vi "test_section_daqmx_task.vi"(8 "error in":errorcluster, 9 "Test Section Physical Channels":T1={"Vapor Mass Flow Current"="cDAQ1Mod1/ai10", "Vapor Line Density Current"="cDAQ1Mod1/ai11", "Liquid Mass Flow Current"="cDAQ1Mod1/ai8", "Liquid Line Density Current"="cDAQ1Mod1/ai9", "Vapor Tank Pressure"="cDAQ1Mod1/ai3", "Liquid Tank Pressure"="cDAQ1Mod1/ai6", "Separator Pressure"="cDAQ1Mod1/ai2", "Liquid Inlet Pressure"="cDAQ1Mod1/ai4", "Vapor Inlet Pressure"="cDAQ1Mod1/ai0", "Vapor Tank Temperature"="cDAQ1Mod1/ai1", "Vapor Inlet Temperature"="cDAQ1Mod6/ai2", "Liquid Tank Temperature"="cDAQ1Mod6/ai0", "Liquid Inlet Temperature"="cDAQ1Mod6/ai3", "Separator Temperature"="cDAQ1Mod6/ai4", "Lower Dev Section Pressure"="cDAQ1Mod6/ai1", "Test Section Temperature"="cDAQ1Mod1/ai5", "Upper Dev Section Temperature"="cDAQ1Mod1/ai12", "Upper Dev Section Pressure"="cDAQ1Mod6/ai9", "Atmospheric Pressure"="cDAQ1Mod5/ai7", "Mixing Tee dP"="cDAQ1Mod6/ai5", "PG inlet-Mixing Tee Pressure"="cDAQ1Mod6/ai5", "Test Section Pressure"="cDAQ1Mod5/ai7", "PG inlet-Mixing Tee Temperature"="cDAQ1Mod6/ai5"}) -> (0 "error out":errorcluster, 3 "task out":refnum<k21>)   [LabVIEW 2017]
uses:
  Input Channel Lists/test_section_physical_channels.ctl
  <vilib>/DAQmx/create/channels.llb/DAQmx Create Channel (AI-Current-Basic).vi
  <vilib>/DAQmx/create/channels.llb/DAQmx Create Channel (AI-Voltage-Basic).vi
  <vilib>/DAQmx/create/channels.llb/DAQmx Create Channel (AI-Temperature-Thermocouple).vi
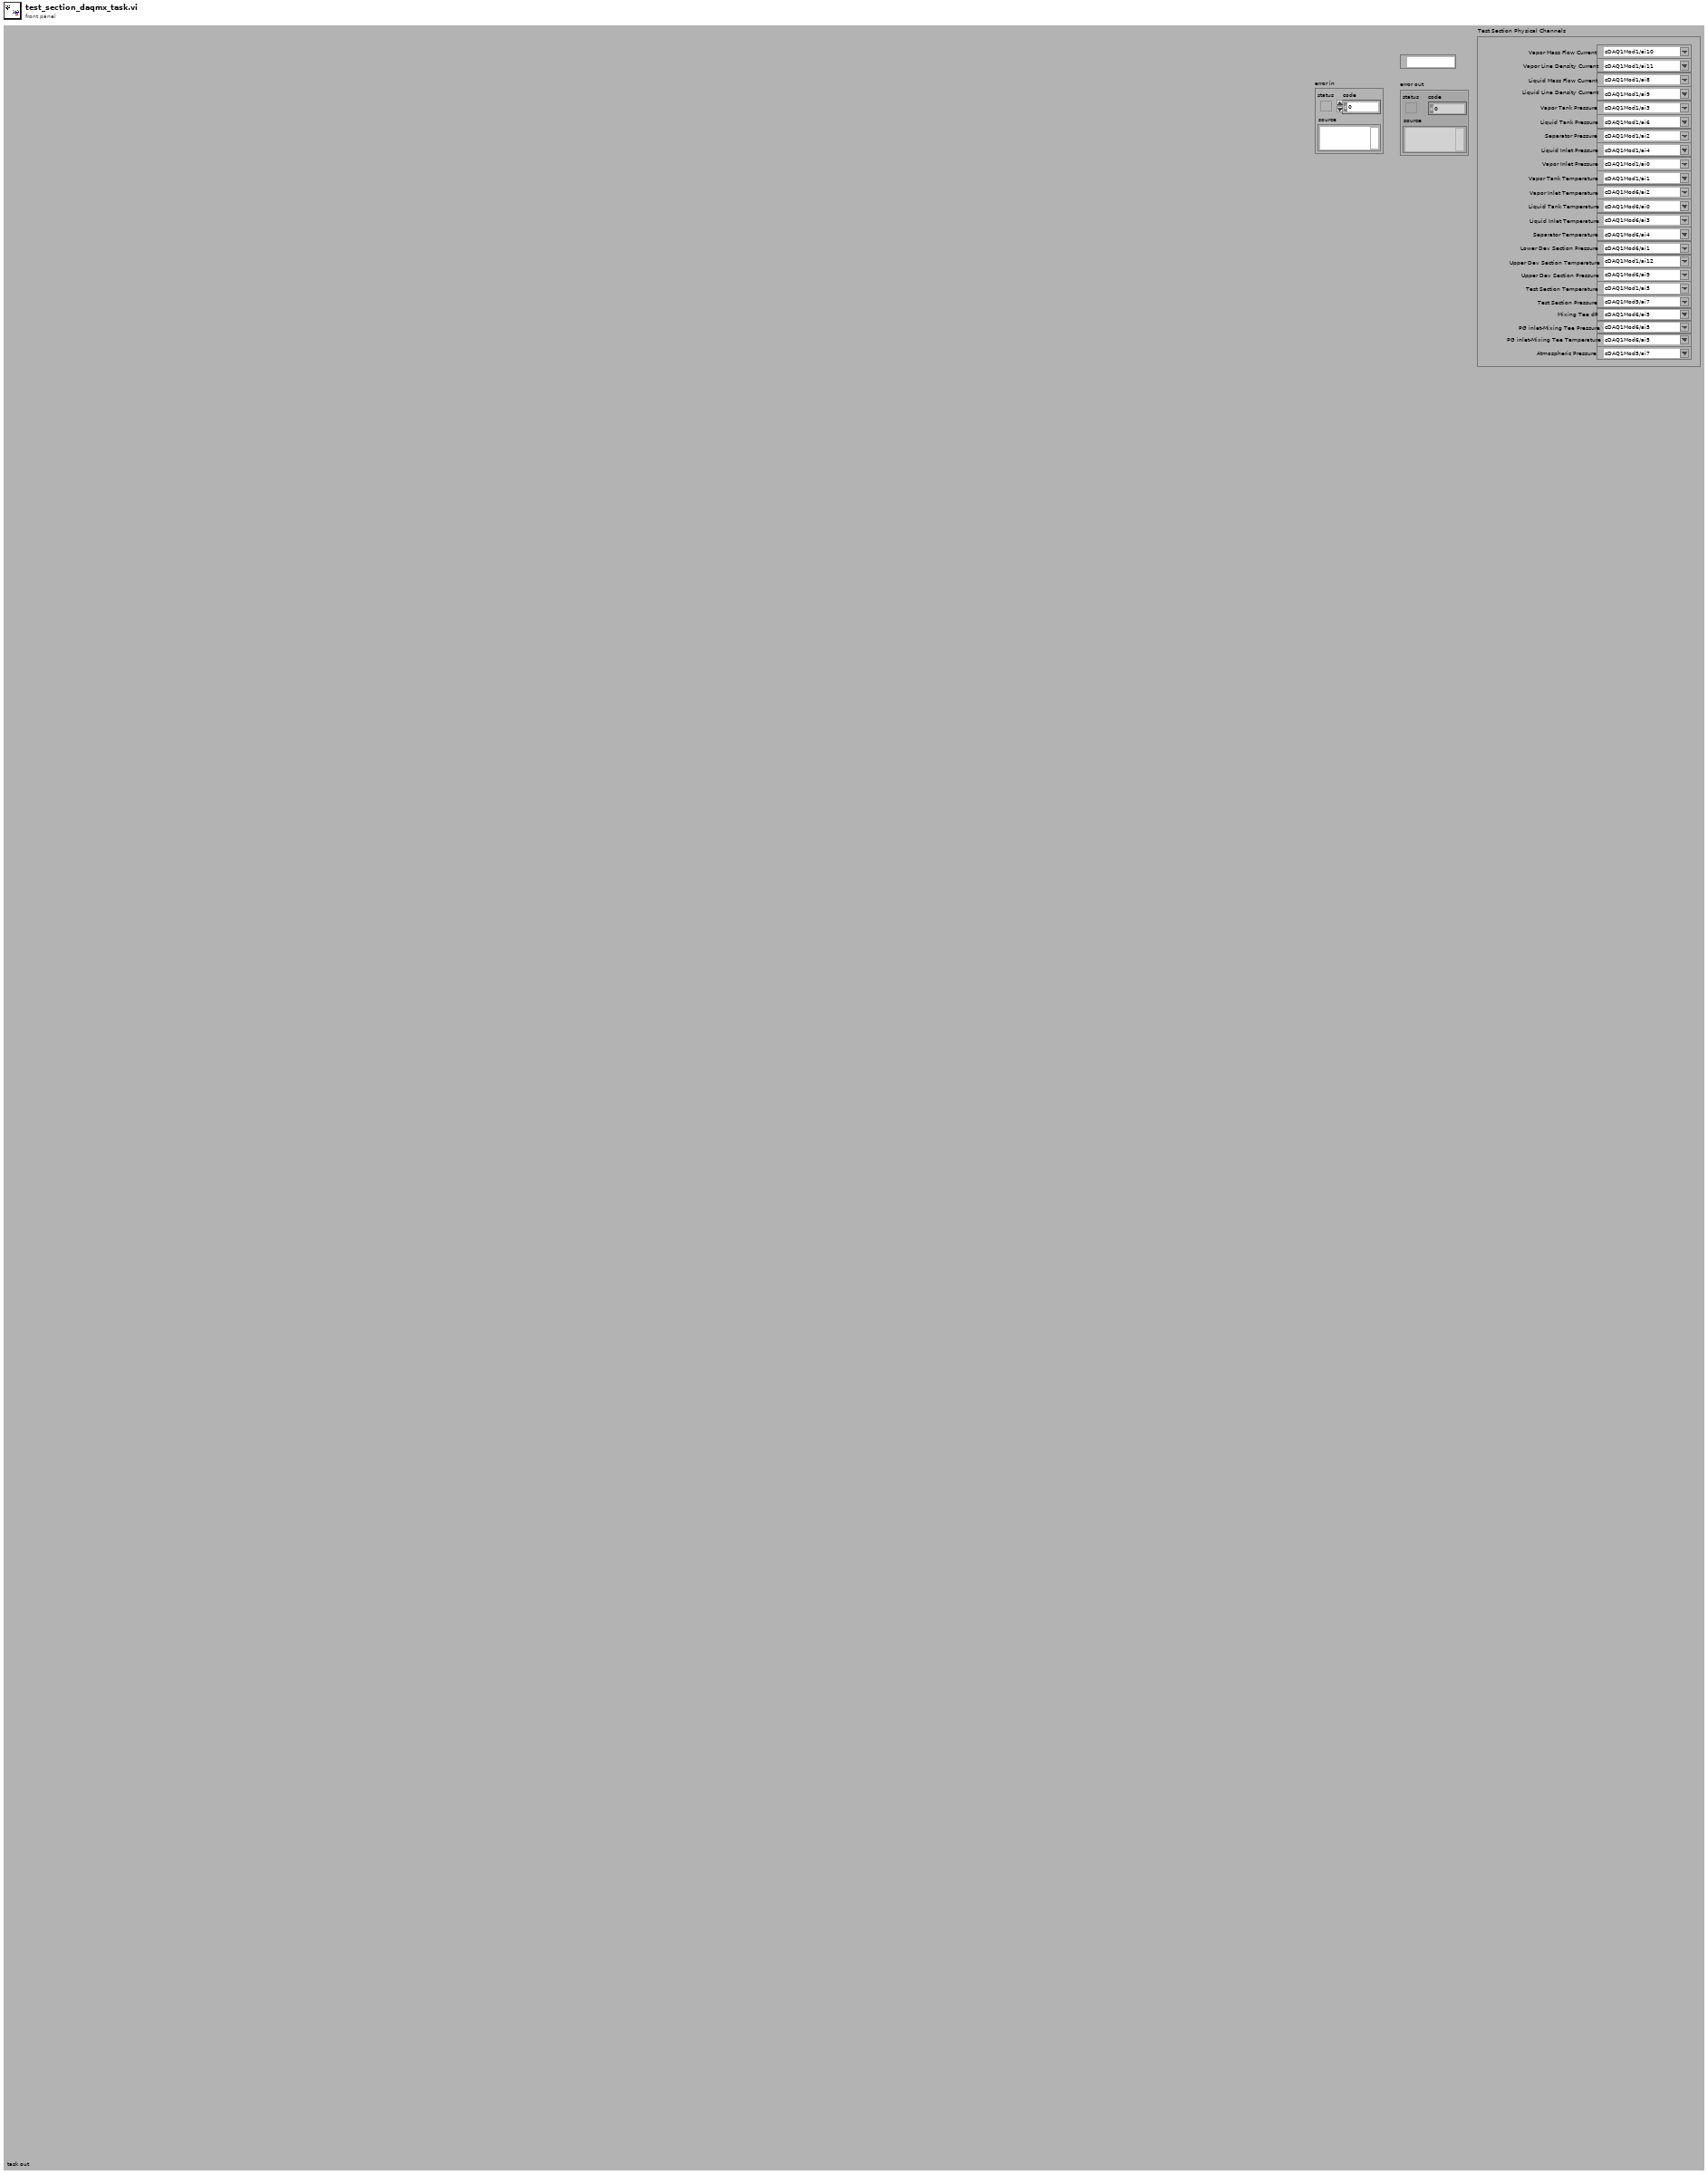
[diagram p1: front panel]
types:
  T1 = typedef "test_section_physical_channels.ctl" = cluster{"Vapor Mass Flow Current":tag, "Vapor Line Density Current":tag, "Liquid Mass Flow Current":tag, "Liquid Line Density Current":tag, "Vapor Tank Pressure":tag, "Liquid Tank Pressure":tag, "Separator Pressure":tag, "Liquid Inlet Pressure":tag, "Vapor Inlet Pressure":tag, "Vapor Tank Temperature":tag, "Vapor Inlet Temperature":tag, "Liquid Tank Temperature":tag, "Liquid Inlet Temperature":tag, "Separator Temperature":tag, "Lower Dev Section Pressure":tag, "Test Section Temperature":tag, "Upper Dev Section Temperature":tag, "Upper Dev Section Pressure":tag, "Atmospheric Pressure":tag, "Mixing Tee dP":tag, "PG inlet-Mixing Tee Pressure":tag, "Test Section Pressure":tag, "PG inlet-Mixing Tee Temperature":tag}
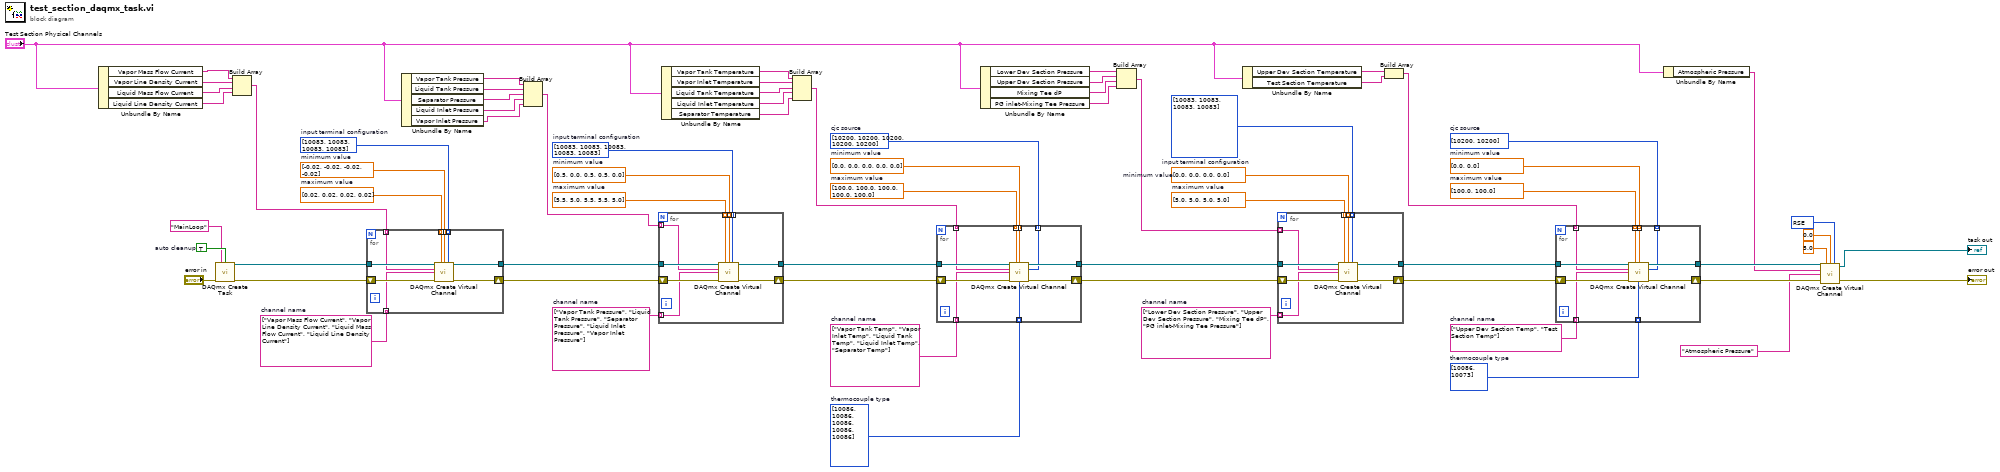
[diagram p0: block diagram]
diagram:
  w4 = 10083 items=["Default"=-1, "RSE"=10083, "NRSE"=10078, "Differential"=10106, "Pseudodifferential"=12529] ("input terminal configuration")
  w39 = i32[] [10086, 10073] items=["J"=10072, "K"=10073, "N"=10077, "R"=10082, "S"=10085, "T"=10086, "B"=10047, "E"=10055]  # thermocouple type
  w38 = string[] ["Upper Dev Section Temp", "Test Section Temp"]  # channel name
  w40 = dbl[] [100.0, 100.0]  # maximum value
  w41 = dbl[] [0.0, 0.0]  # minimum value
  w37 = u32[] [10200, 10200] items=["Internal"=10200, "Constant Value"=10116, "Channel"=10113]  # cjc source
  w44 = string[] ["Lower Dev Section Pressure", "Upper Dev Section Pressure", "Mixing Tee dP", "PG inlet-Mixing Tee Pressure"]  # channel name
  w45 = dbl[] [5.0, 5.0, 5.0, 5.0]  # maximum value
  w46 = dbl[] [0.0, 0.0, 0.0, 0.0]  # minimum value
  w47 = i32[] [10083, 10083, 10083, 10083] items=["default"=-1, "RSE"=10083, "NRSE"=10078, "Differential"=10106, "Pseudodifferential"=12529]  # input terminal configuration
  w52 = i32[] [10086, 10086, 10086, 10086, 10086] items=["J"=10072, "K"=10073, "N"=10077, "R"=10082, "S"=10085, "T"=10086, "B"=10047, "E"=10055]  # thermocouple type
  w51 = string[] ["Vapor Tank Temp", "Vapor Inlet Temp", "Liquid Tank Temp", "Liquid Inlet Temp", "Separator Temp"]  # channel name
  w53 = dbl[] [100.0, 100.0, 100.0, 100.0, 100.0]  # maximum value
  w54 = dbl[] [0.0, 0.0, 0.0, 0.0, 0.0]  # minimum value
  w49 = u32[] [10200, 10200, 10200, 10200, 10200] items=["Internal"=10200, "Constant Value"=10116, "Channel"=10113]  # cjc source
  w57 = string[] ["Vapor Tank Pressure", "Liquid Tank Pressure", "Separator Pressure", "Liquid Inlet Pressure", "Vapor Inlet Pressure"]  # channel name
  w58 = dbl[] [5.5, 5.0, 5.5, 5.5, 5.0]  # maximum value
  w59 = dbl[] [0.5, 0.0, 0.5, 0.5, 0.0]  # minimum value
  w60 = i32[] [10083, 10083, 10083, 10083, 10083] items=["default"=-1, "RSE"=10083, "NRSE"=10078, "Differential"=10106, "Pseudodifferential"=12529]  # input terminal configuration
  w63 = string[] ["Vapor Mass Flow Current", "Vapor Line Density Current", "Liquid Mass Flow Current", "Liquid Line Density Current"]  # channel name
  w64 = dbl[] [0.02, 0.02, 0.02, 0.02]  # maximum value
  w65 = dbl[] [-0.02, -0.02, -0.02, -0.02]  # minimum value
  w66 = i32[] [10083, 10083, 10083, 10083] items=["default"=-1, "RSE"=10083, "NRSE"=10078, "Differential"=10106, "Pseudodifferential"=12529]  # input terminal configuration
  w68 = TRUE  # auto cleanup
  n1 = Unbundle By Name("Test Section Physical Channels") -> ("Vapor Mass Flow Current"=w35:tag, "Vapor Line Density Current"=w34:tag, "Liquid Mass Flow Current"=w33:tag, "Liquid Line Density Current"=w32:tag)
  n2 = call <vilib>:"DAQmx Create Task.vi"("new task name"="MainLoop", "auto cleanup"=w68, "error in"="error in") -> ("task out"=w67:refnum<k21>, "error out"=w69:errorcluster)  [unwired: 11 in]
  n3 = Build Array(w35, w34, w33, w32) -> (w31:tag[])
  n4 = for {
    tunnel: w67 -> [w76]
    tunnel: w66 -> [w79] mode=indexing
    tunnel: w65 -> [w78] mode=indexing
    tunnel: w64 -> [w77] mode=indexing
    tunnel: w63 -> [w72] mode=indexing
    tunnel: w31 -> [w71] mode=indexing
    tunnel: [w74] -> w61
    shift-right: [w73] -> w62
    shift-left: w69 -> [w75]
    n5 = call-poly <vilib>:"DAQmx Create Virtual Channel.vi"("task in"=w76, "maximum value"=w77, "minimum value"=w78, "input terminal configuration"=w79, "physical channels"=w71, "name to assign"=w72, "error in"=w75) -> ("task out"=w74:refnum<k21>, "error out"=w73:errorcluster)  [unwired: 7 in]
  }
  n6 = Unbundle By Name("Test Section Physical Channels") -> ("Vapor Tank Pressure"=w27:tag, "Liquid Tank Pressure"=w28:tag, "Separator Pressure"=w29:tag, "Liquid Inlet Pressure"=w30:tag, "Vapor Inlet Pressure"=w21:tag)
  n7 = Build Array(w27, w28, w29, w30, w21) -> (w20:tag[])
  n8 = for {
    tunnel: w61 -> [w85]
    tunnel: w60 -> [w86] mode=indexing
    tunnel: w59 -> [w87] mode=indexing
    tunnel: w58 -> [w88] mode=indexing
    tunnel: w57 -> [w81] mode=indexing
    tunnel: w20 -> [w80] mode=indexing
    tunnel: [w83] -> w55
    shift-right: [w82] -> w56
    shift-left: w62 -> [w84]
    n9 = call-poly <vilib>:"DAQmx Create Virtual Channel.vi"("task in"=w85, "maximum value"=w88, "minimum value"=w87, "input terminal configuration"=w86, "physical channels"=w80, "name to assign"=w81, "error in"=w84) -> ("task out"=w83:refnum<k21>, "error out"=w82:errorcluster)  [unwired: 7 in]
  }
  n10 = Unbundle By Name("Test Section Physical Channels") -> ("Vapor Tank Temperature"=w26:tag, "Vapor Inlet Temperature"=w25:tag, "Liquid Tank Temperature"=w24:tag, "Liquid Inlet Temperature"=w23:tag, "Separator Temperature"=w19:tag)
  n11 = Build Array(w26, w25, w24, w23, w19) -> (w18:tag[])
  n12 = for {
    tunnel: w55 -> [w96]
    tunnel: w54 -> [w97] mode=indexing
    tunnel: w53 -> [w98] mode=indexing
    tunnel: w52 -> [w89] mode=indexing
    tunnel: w51 -> [w92] mode=indexing
    tunnel: w18 -> [w91] mode=indexing
    tunnel: [w94] -> w48
    tunnel: w49 -> [w90] mode=indexing
    shift-right: [w93] -> w50
    shift-left: w56 -> [w95]
    n13 = call-poly <vilib>:"DAQmx Create Virtual Channel.vi"("task in"=w96, "maximum value"=w98, "minimum value"=w97, "physical channels"=w91, "cjc source"=w90, "name to assign"=w92, "error in"=w95, "thermocouple type"=w89) -> ("task out"=w94:refnum<k21>, "error out"=w93:errorcluster)  [unwired: 6 in]
  }
  n14 = Unbundle By Name("Test Section Physical Channels") -> ("Lower Dev Section Pressure"=w22:tag, "Upper Dev Section Pressure"=w14:tag, "Mixing Tee dP"=w2:tag, "PG inlet-Mixing Tee Pressure"=w1:tag)
  n15 = Build Array(w22, w14, w2, w1) -> (w17:tag[])
  n16 = Unbundle By Name("Test Section Physical Channels") -> ("Upper Dev Section Temperature"=w16:tag, "Test Section Temperature"=w13:tag)
  n17 = for {
    tunnel: w48 -> [w104]
    tunnel: w47 -> [w105] mode=indexing
    tunnel: w46 -> [w106] mode=indexing
    tunnel: w45 -> [w107] mode=indexing
    tunnel: w44 -> [w100] mode=indexing
    tunnel: w17 -> [w99] mode=indexing
    tunnel: [w102] -> w42
    shift-right: [w101] -> w43
    shift-left: w50 -> [w103]
    n18 = call-poly <vilib>:"DAQmx Create Virtual Channel.vi"("task in"=w104, "maximum value"=w107, "minimum value"=w106, "input terminal configuration"=w105, "physical channels"=w99, "name to assign"=w100, "error in"=w103) -> ("task out"=w102:refnum<k21>, "error out"=w101:errorcluster)  [unwired: 7 in]
  }
  n19 = Build Array(w16, w13) -> (w15:tag[])
  n20 = for {
    tunnel: w42 -> [w115]
    tunnel: w41 -> [w116] mode=indexing
    tunnel: w40 -> [w117] mode=indexing
    tunnel: w39 -> [w108] mode=indexing
    tunnel: w38 -> [w111] mode=indexing
    tunnel: w15 -> [w110] mode=indexing
    tunnel: [w113] -> w12
    tunnel: w37 -> [w109] mode=indexing
    shift-right: [w112] -> w11
    shift-left: w43 -> [w114]
    n21 = call-poly <vilib>:"DAQmx Create Virtual Channel.vi"("task in"=w115, "maximum value"=w117, "minimum value"=w116, "physical channels"=w110, "cjc source"=w109, "name to assign"=w111, "error in"=w114, "thermocouple type"=w108) -> ("task out"=w113:refnum<k21>, "error out"=w112:errorcluster)  [unwired: 6 in]
  }
  n22 = Unbundle By Name("Test Section Physical Channels") -> ("Atmospheric Pressure"=w7:tag)
  n23 = call-poly <vilib>:"DAQmx Create Virtual Channel.vi"("task in"=w12, "maximum value"=5.0, "minimum value"=0.0, "input terminal configuration"=w4, "physical channels"=w7, "name to assign"="Atmospheric Pressure", "error in"=w11) -> ("task out"=→"task out":refnum<k21>, "error out"=→"error out":errorcluster)  [unwired: 7 in]
